vi "5.10 Exposure.vi"(1 "Session In":T1, 2 "Exposure":dbl) -> (0 "Session Out":T1)   [LabVIEW 2010]
uses:
  <vilib>/userDefined/High Color/IMAQdx.ctl
  Program Files (x86)/National Instruments/LabVIEW 2010/resource/objmgr/imaqdx.rc
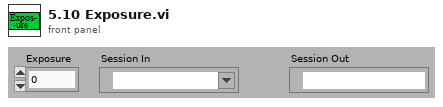
[diagram p1: front panel]
types:
  T1 = typedef "IMAQdx.ctl" = refnum<k21>
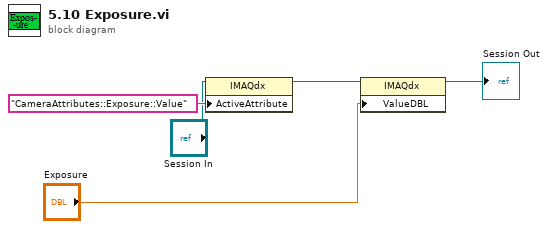
[diagram p0: block diagram]
diagram:
  n1 = property class="IMAQdx"(reference="Session In", "ActiveAttribute"="CameraAttributes::Exposure::Value") -> (reference out=w3:T1)  [unwired: 1 in, 1 out]
  n2 = property class="IMAQdx"(reference=w3, "ValueDBL"="Exposure") -> (reference out=→"Session Out":T1)  [unwired: 1 in, 1 out]
